vi "trigger_digitimer.vi"(7 "data":waveform(dbl)={"t0"=timestamp(0 s since 1904-01-01), "dt"=0.0, "Y"=[]}, 8 "error in":errorcluster, 10 "trigger samples":i32, 11 "physical channels":tag) -> (0 "error out":errorcluster, 3 "SampClk.Rate":dbl)   [LabVIEW 2020]
uses:
  <vilib>/DAQmx/write.llb/DAQmx Write (Analog Wfm 1Chan NSamp).vi
  <vilib>/DAQmx/create/channels.llb/DAQmx Create Channel (AO-Voltage-Basic).vi
  <vilib>/DAQmx/configure/timing.llb/DAQmx Timing (Sample Clock).vi
  <resource>/objmgr/daqmx.rc
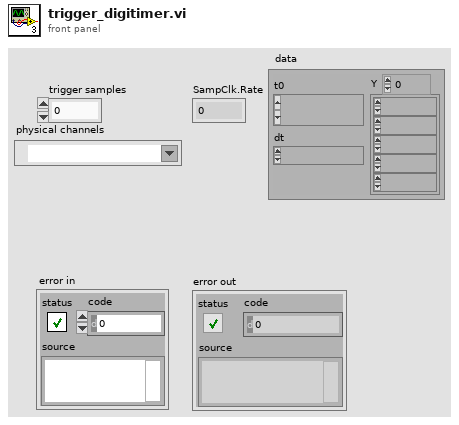
[diagram p1: front panel]
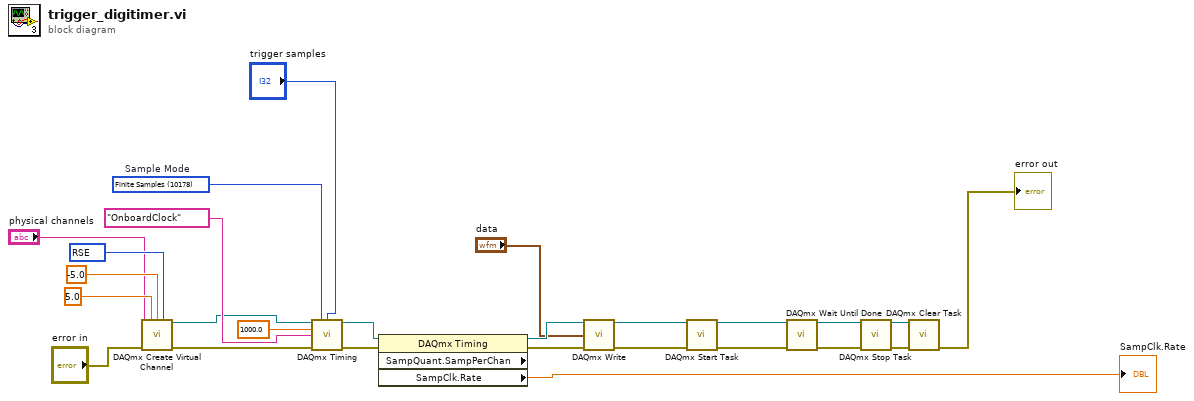
[diagram p0: block diagram]
diagram:
  w24 = 10083 items=["Default"=-1, "RSE"=10083, "Differential"=10106, "Pseudodifferential"=12529] ("output terminal configuration")
  w14 = 10178 items=["Finite Samples"=10178, "Continuous Samples"=10123, "Hardware Timed Single Point"=12522]  # Sample Mode
  n1 = call-poly <vilib>:"DAQmx Create Virtual Channel.vi"("maximum value"=5.0 ("Max Voltage"), "minimum value"=-5.0 ("Min Voltage"), "output terminal configuration"=w24, "physical channels"="physical channels", "error in"="error in") -> ("task out"=w16:refnum<k21>, "error out"=w15:errorcluster)  [unwired: 9 in]
  n2 = call-poly <vilib>:"DAQmx Timing.vi"("task/channels in"=w16, "sample mode"=w14, "samples per channel"="trigger samples", "rate"=1000.0 ("Sample Rate"), "source"=tag "OnboardClock" ("Sample Clock Source"), "error in"=w15) -> ("task out"=w12:refnum<k21>, "error out"=w13:errorcluster)  [unwired: 8 in]
  n3 = property class="DAQmx Timing" props=["SampQuant.SampPerChan", "SampClk.Rate"](reference=w12, error in=w13) -> (reference out=w21:refnum<k21>, error out=w22:errorcluster, "SampClk.Rate"=→"SampClk.Rate":dbl)  [unwired: 1 out]
  n4 = call-poly <vilib>:"DAQmx Write.vi"("task/channels in"=w21, "data"="data", "error in"=w22) -> ("task out"=w11:refnum<k21>, "error out"=w10:errorcluster)  [unwired: 10 in, 1 out]
  n5 = call <vilib>:"DAQmx Start Task.vi"("task/channels in"=w11, "error in"=w10) -> ("task out"=w9:refnum<k21>, "error out"=w8:errorcluster)  [unwired: 12 in]
  n6 = call <vilib>:"DAQmx Wait Until Done.vi"("task/channels in"=w9, "error in"=w8) -> ("task out"=w5:refnum<k21>, "error out"=w4:errorcluster)  [unwired: 12 in]
  n7 = call <vilib>:"DAQmx Stop Task.vi"("task/channels in"=w5, "error in"=w4) -> ("task out"=w7:refnum<k21>, "error out"=w6:errorcluster)  [unwired: 12 in]
  n8 = call <vilib>:"DAQmx Clear Task.vi"("task in"=w7, "error in"=w6) -> ("error out"=→"error out":errorcluster)  [unwired: 13 in]
